vi "Create Default Configuration.vi"(0 "Sinks":refnum<class "Sink.lvclass">[](array[class]), 2 "Debug Level in":T1=enum."DEBUG", 3 "error in (no error)":errorcluster) -> (10 "error out":errorcluster)   [LabVIEW 2020, in "LV Log.lvlib"]
uses:
  LV Log.lvlib
  Type Defs/Debug Level.ctl
  Sinks/Sink/Sink.lvclass
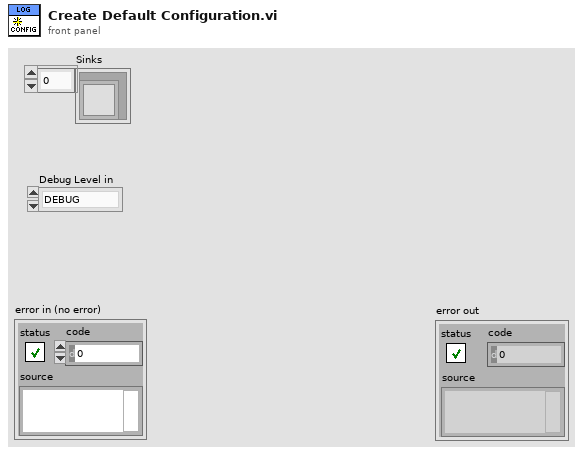
[diagram p1: front panel]
types:
  T1 = typedef "LV Log.lvlib/Debug Level.ctl" = enum16{"DEFAULT", "DEBUG", "INFO", "WARN", "ERROR", "FATAL"}
  T2 = enum16{"Init", "Get Logger", "Register Sink", "Set Global Debug Level", "Get Sinks", "Get Global Debug Level", "Register Logger"}
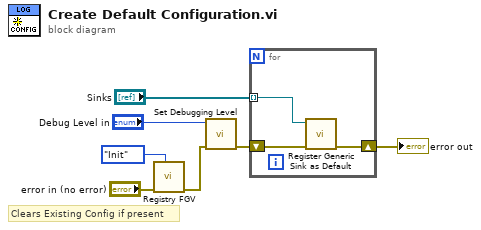
[diagram p0: block diagram]
diagram:
  # "Clears Existing Config if present"
  n1 = call "Registry FGV.vi"("State (Get Logger)"=T2."Init", "error in (no error)"="error in (no error)") -> ("error out"=w3:errorcluster)  [unwired: 6 in, 3 out]
  n2 = call "Set Debugging Level.vi"("error in (no error)"=w3, "Debug Level in"="Debug Level in") -> ("error out"=w7:errorcluster)  [unwired: 9 in]
  n3 = for {
    tunnel: "Sinks" -> [w8] mode=indexing
    shift-right: [w9] -> w6
    shift-left: w7 -> [w10]
    n4 = call "Register Generic Sink as Default.vi"("error in (no error)"=w10, "Sink"=w8) -> ("error out"=w9:errorcluster)  [unwired: 9 in]
  }
  "error out" <- w6
